vi "camera acquire test.vi"() -> ()   [LabVIEW 2014]
uses:
  SubVIs/ctt's/image acquisiton 4.ctl
  SubVIs/ctt's/image acquisition 3.ctl
  <vilib>/vision/Image Controls.llb/IMAQ Image.ctl
  SubVIs/Initilize Globals.vi
  lib/Andorlib/atmcd32d.lvlib
panel:
  out "Error Out":errorcluster
  out "Image Out":T1
  in  "Image In":T1
  out "Error Return":i32
  in  "High Capacity?":bool
  in  "Acquisition Parameters":T2={"Readout Mode"=enum."Image", "Set Acquisition Mode"=enum."Single Scan", "Trigger Mode"=enum."Internal", "Exposure Time (s)"=1.0, "Accumulation Cycle (s)"=1.0, "Kinetic Cycle Time (s)"=1.0, "Number of Kinetics"=1, "Number of Accumulations"=1, "Set VS Speed"=1, "Pixel Rate"=enum."Standard CCD 3 Mhz 14 bits", "V Shift Amplitude"=enum."+1", "Preamp Gain"=enum."1.0"}
  in  "Image Size":T3={"H Bin"=1024.0, "V Bin"=1024.0, "Left"=1.0, "Right"=1024.0, "Top"=1.0, "Bottom"=1024.0} {"V Bin" min=0.0; "H Bin" min=0.0 step=1.0}
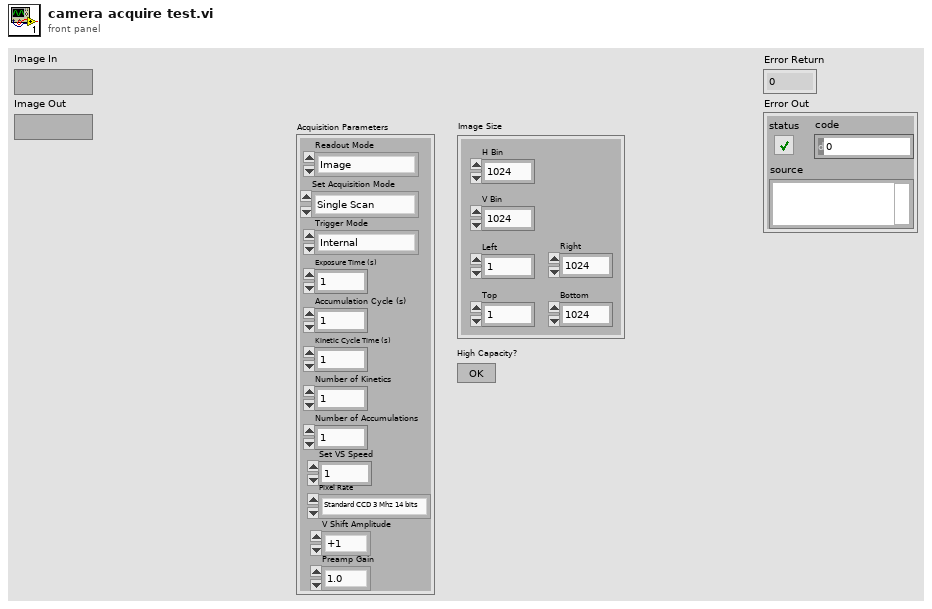
[diagram p1: front panel]
types:
  T1 = typedef "IMAQ Image.ctl" = refnum<image>
  T2 = typedef "image acquisition 3.ctl" = cluster{"Readout Mode":enum16{"Full Vertical Binning", "Multi-Track", "Random-Track", "Single-Track", "Image"}, "Set Acquisition Mode":enum16{"(do nothing)", "Single Scan", "Accumulate", "Kinetics", "Fast Kinetics", "Run till abort"}, "Trigger Mode":enum16{"Internal", "External"}, "Exposure Time (s)":dbl, "Accumulation Cycle (s)":dbl, "Kinetic Cycle Time (s)":dbl, "Number of Kinetics":i32, "Number of Accumulations":i32, "Set VS Speed":i32, "Pixel Rate":enum16{"EM CCD 10 Mhz 14 bits", "EM CCD 5 Mhz 14 bits", "EM CCD 3 Mhz 14 bits", "EM CCD 1 Mhz 16 bits", "Standard CCD 3 Mhz 14 bits", "Standard CCD 1 Mhz 16 bits"}, "V Shift Amplitude":enum16{"normal", "+1", "+2", "+3", "+4"}, "Preamp Gain":enum16{"1.0", "2.4", "5.0"}}
  T3 = typedef "image acquisiton 4.ctl" = cluster{"H Bin":dbl, "V Bin":dbl, "Left":dbl, "Right":dbl, "Top":dbl, "Bottom":dbl}
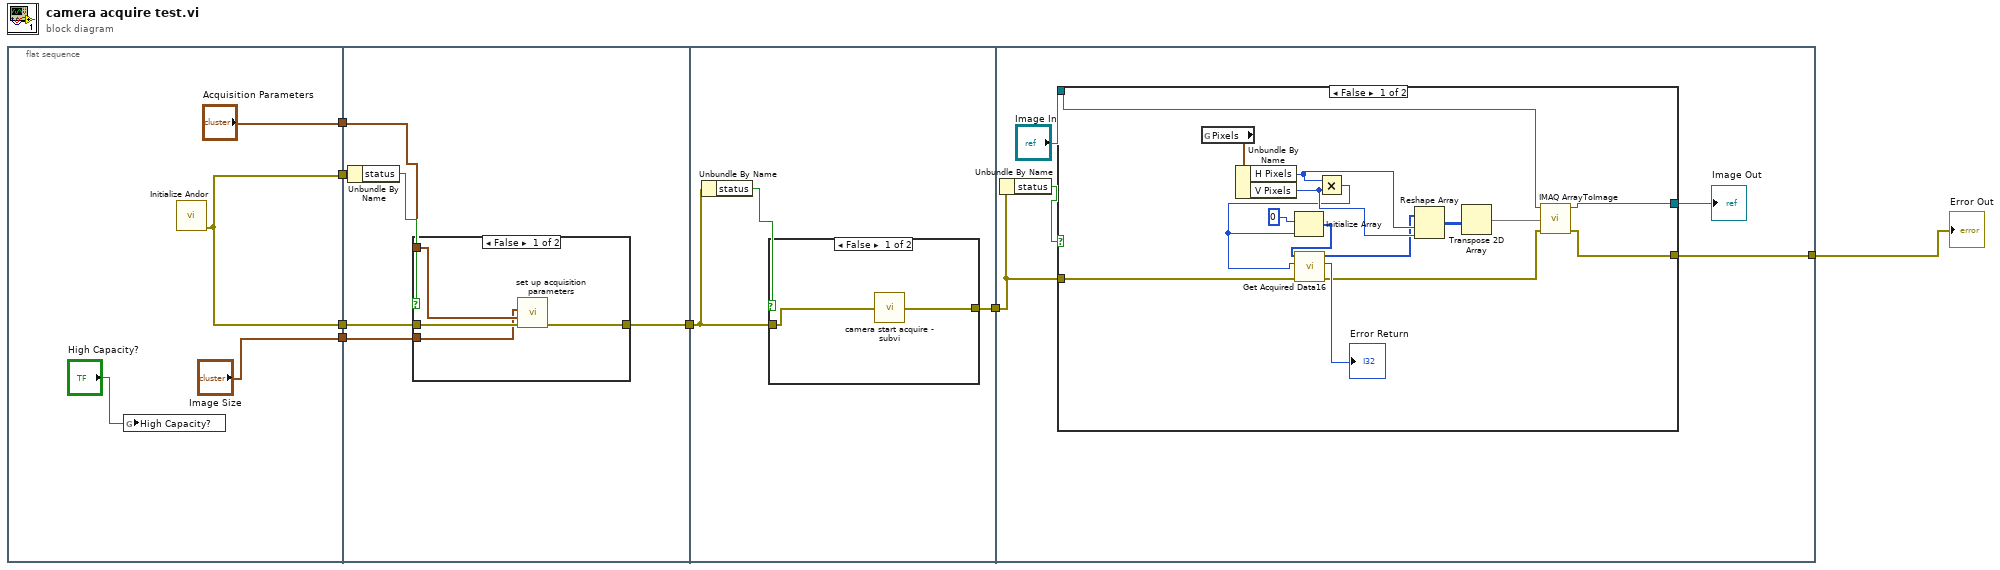
[diagram p0: block diagram]
diagram:
  n1 = flat-sequence {
    tunnel: [w11] -> w7
    tunnel: [w11] -> w6
    tunnel: ["Acquisition Parameters"] -> w3
    tunnel: ["Image Size"] -> w2
    tunnel: w7 -> [w17]
    tunnel: w6 -> [w15]
    tunnel: [w14] -> w5
    tunnel: w3 -> [w13]
    tunnel: w2 -> [w12]
    tunnel: w5 -> [w24]
    tunnel: [w23] -> w4
    tunnel: w4 -> [w33]
    tunnel: [w29] -> w1
    frame #0 {
      n2 = global write "Initilize Globals.vi" "High Capacity?"("High Capacity?") -> ()
      n3 = call "Initialize Andor.vi"() -> ("Error Out 2"=w11:errorcluster)  [unwired: 11 in]
    }
    frame #1 {
      n4 = Unbundle By Name(w17) -> ("status"=w16:bool)
      n5 = case shown="False" w16 {
        tunnel: w15 -> [w21 w22]
        tunnel: [w20 w22] -> w14
        tunnel: w13 -> [w19 _]
        tunnel: w12 -> [w18 _]
        frame False {
          n6 = call "set up acquisition parameters.vi"("error in (no error)"=w21, "Acquisition Parameters"=w19, "Image Size"=w18) -> ("error out"=w20:errorcluster)  [unwired: 2 in, 4 out]
        }
        frame True {
        }
      }
    }
    frame #2 {
      n7 = Unbundle By Name(w24) -> ("status"=w25:bool)
      n8 = case shown="False" w25 {
        tunnel: w24 -> [w27 w28]
        tunnel: [w26 w28] -> w23
        frame False {
          n9 = call "camera start acquire - subvi.vi"("error in"=w27) -> ("error out"=w26:errorcluster)
        }
        frame True {
        }
      }
    }
    frame #3 {
      n10 = Unbundle By Name(w33) -> ("status"=w32:bool)
      n11 = case shown="False" w32 {
        tunnel: w33 -> [w47 w49]
        tunnel: "Image In" -> [w37 w50]
        tunnel: [w36 w50] -> w30
        tunnel: [w35 w49] -> w29
        frame False {
          n12 = global read "Initilize Globals.vi" "Pixels"() -> (w48:cluster{"H Pixels":u32, "V Pixels":u32})
          n13 = Unbundle By Name(w48) -> ("H Pixels"=w43:u32, "V Pixels"=w42:u32)
          n14 = Multiply(x=w43, y=w42) -> (x*y=w34:u32)
          n15 = Initialize Array(u16 0, w34) -> (w45:u16[])
          n16 = call "Get Acquired Data16.vi"("error in (no error)"=w47, "size"=w34, "arr in"=w45) -> ("error out"=w38:errorcluster, "function return"=→"Error Return":u32, "arr out"=w41:u16[])  [unwired: 6 in]
          n17 = Reshape Array(w41, w43, w42) -> (w40:u16[][])
          n18 = Transpose 2D Array(2D array=w40) -> (transposed array=w39:u16[][])
          n19 = call "IMAQ ArrayToImage"("error in (no error)"=w38, "Image Pixels (I16)"=w39, "Image"=w37) -> ("error out"=w35:errorcluster, "Image Out"=w36:T1)  [unwired: 3 in, 4 out]
        }
        frame True {
        }
      }
      "Image Out" <- w30
    }
  }
  "Error Out" <- w1
